vi "4155C Config V Stress v2.0.vi"(1 "Display on/off":bool, 2 "Stress V - Gate":u32(ring)=2 items=["SMU1  ", "SMU2  ", "SMU3  ", "SMU4  ", "SMU5  ", "SMU6  "], 4 "Stress V - Drain":u32(ring)=1 items=["SMU1  ", "SMU2  ", "SMU3  ", "SMU4  ", "SMU5  ", "SMU6  "], 5 "Stress V - Source/Common":u32(ring) items=["SMU1  ", "SMU2  ", "SMU3  ", "SMU4  ", "SMU5  ", "SMU6  "], 6 "IG compliance":dbl min=0.0 max=100000000000.0 format="%.15e", 7 "ID compliance":dbl min=0.0 max=100000000000.0 format="%.15e", 8 "error in (no error)":errorcluster, 9 "VG":dbl min=0.0 max=100000000000.0 format="%.15e", 10 "VD":dbl min=0.0 max=100000000000.0 format="%.15e", 11 "VISA session":refnum<visa-resource-name>) -> (0 "error out":errorcluster, 3 "dup VISA resource name":refnum<visa-resource-name>)   [LabVIEW 2016]
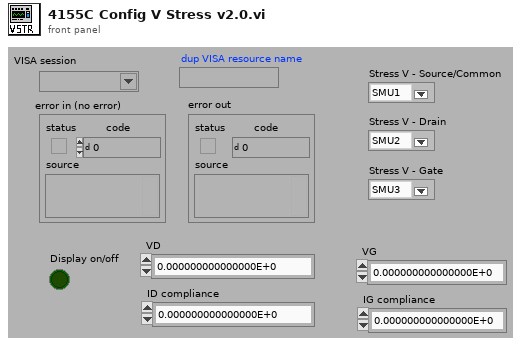
[diagram p1: front panel]
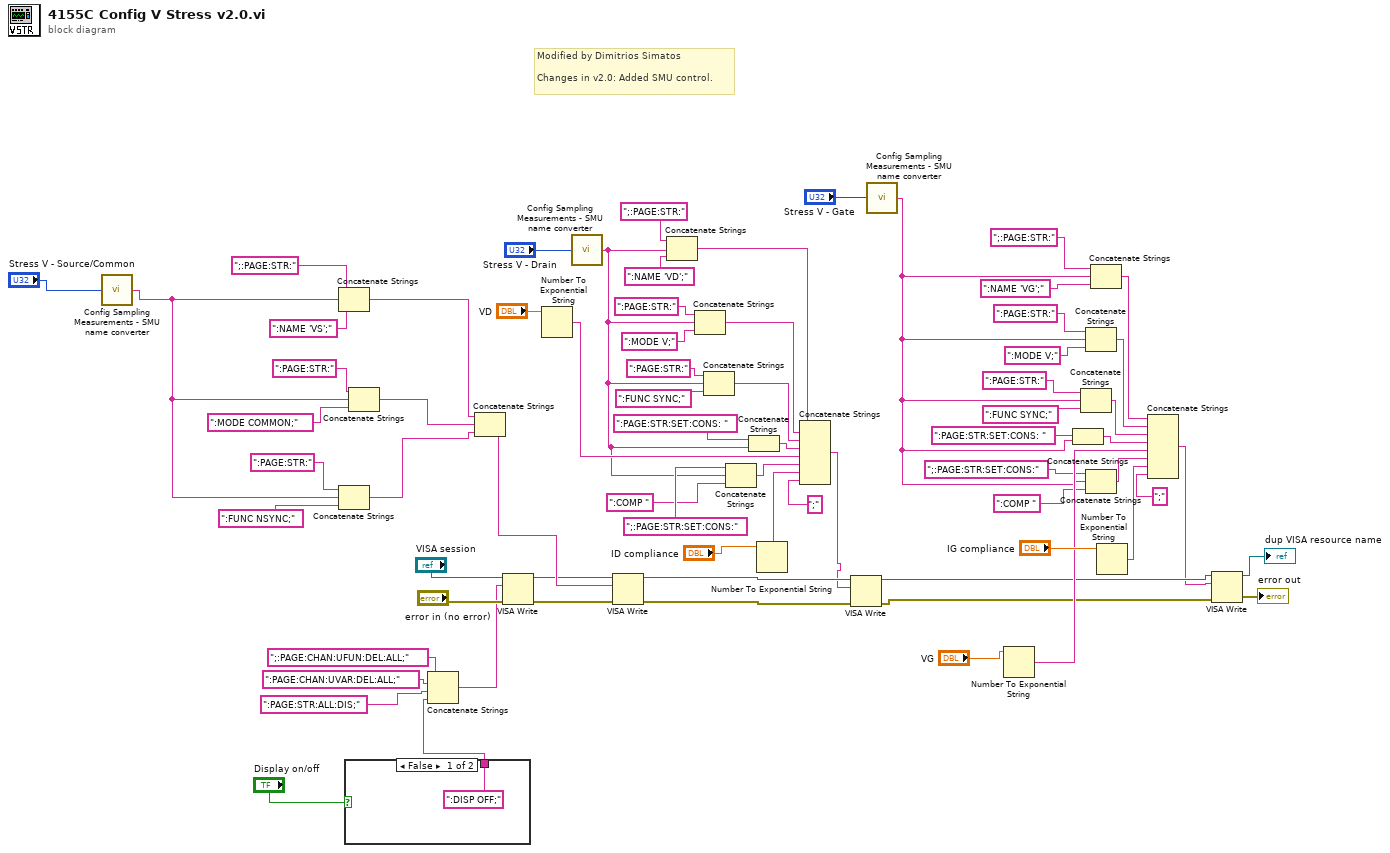
[diagram p0: block diagram]
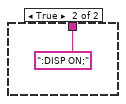
[diagram p2: hidden frame]
diagram:
  # "Modified by Dimitrios Simatos\n\nChanges in v2.0: Added SMU control."
  n1 = call "Config Sampling Measurements - SMU name converter.vi"("unit to configure"="Stress V - Source/Common") -> ("SMU to be configured"=w41:string)
  n2 = Concatenate Strings(";:PAGE:STR:", w41, ":NAME 'VS';") -> (w40:string)
  n3 = Concatenate Strings(":PAGE:STR:", w41, ":FUNC NSYNC;") -> (w38:string)
  n4 = case shown="False" "Display on/off" {
    tunnel: [":DISP OFF;" ("write buffer (\"\")") ":DISP ON;" ("write buffer (\"\")")] -> w66
    frame False {
    }
    frame True {
    }
  }
  n5 = Concatenate Strings(":PAGE:STR:", w41, ":MODE COMMON;") -> (w39:string)
  n6 = Concatenate Strings(";:PAGE:CHAN:UFUN:DEL:ALL;", ":PAGE:CHAN:UVAR:DEL:ALL;", ":PAGE:STR:ALL:DIS;", w66) -> (w67:string)
  n7 = Concatenate Strings(w40, w39, w38) -> (w52:string)
  n8 = VISA Write(VISA resource name="VISA session", write buffer=w67, error in (no error)="error in (no error)") -> (VISA resource name out=w51:refnum<visa-resource-name>, error out=w50:errorcluster)  [unwired: 1 out]
  n9 = Number To Exponential String(number="VD") -> (E-format string=w60:string)  [unwired: 3 in]
  n10 = call "Config Sampling Measurements - SMU name converter.vi"("unit to configure"="Stress V - Drain") -> ("SMU to be configured"=w17:string)
  n11 = VISA Write(VISA resource name=w51, write buffer=w52, error in (no error)=w50) -> (VISA resource name out=w72:refnum<visa-resource-name>, error out=w71:errorcluster)  [unwired: 1 out]
  n12 = Concatenate Strings(";:PAGE:STR:", w17, ":NAME 'VD';") -> (w28:string)
  n13 = Concatenate Strings(":PAGE:STR:", w17, ":MODE V;") -> (w25:string)
  n14 = Concatenate Strings(":PAGE:STR:", w17, ":FUNC SYNC;") -> (w22:string)
  n15 = Concatenate Strings(";:PAGE:STR:SET:CONS:", w17, ":COMP ") -> (w16:string)
  n16 = Concatenate Strings(":PAGE:STR:SET:CONS: ", w17) -> (w20:string)
  n17 = Number To Exponential String(number="ID compliance") -> (E-format string=w58:string)  [unwired: 3 in]
  n18 = Concatenate Strings(w28, w25, w22, w20, w60, w16, w58, ";" ("Substring")) -> (w49:string)
  n19 = VISA Write(VISA resource name=w72, write buffer=w49, error in (no error)=w71) -> (VISA resource name out=w47:refnum<visa-resource-name>, error out=w48:errorcluster)  [unwired: 1 out]
  n20 = call "Config Sampling Measurements - SMU name converter.vi"("unit to configure"="Stress V - Gate") -> ("SMU to be configured"=w1:string)
  n21 = Number To Exponential String(number="VG") -> (E-format string=w55:string)  [unwired: 3 in]
  n22 = Concatenate Strings(":PAGE:STR:SET:CONS: ", w1) -> (w5:string)
  n23 = Concatenate Strings(":PAGE:STR:", w1, ":FUNC SYNC;") -> (w9:string)
  n24 = Concatenate Strings(":PAGE:STR:", w1, ":MODE V;") -> (w12:string)
  n25 = Concatenate Strings(";:PAGE:STR:SET:CONS:", w1, ":COMP ") -> (w4:string)
  n26 = Concatenate Strings(";:PAGE:STR:", w1, ":NAME 'VG';") -> (w13:string)
  n27 = Number To Exponential String(number="IG compliance") -> (E-format string=w53:string)  [unwired: 3 in]
  n28 = Concatenate Strings(w13, w12, w9, w5, w55, w4, w53, ";" ("Substring")) -> (w46:string)
  n29 = VISA Write(VISA resource name=w47, write buffer=w46, error in (no error)=w48) -> (VISA resource name out=→"dup VISA resource name":refnum<visa-resource-name>, error out=→"error out":errorcluster)  [unwired: 1 out]
